vi "User Event LV2.vi"(11 "error in (no error)":errorcluster, 13 "LV2 Mode":T1=enum."Delete") -> (4 "Stop Val":refnum<user-event>, 15 "error out":errorcluster)   [LabVIEW 2020, in "I2C Controller Lib.lvlib"]
doc: "User events LV2 used to Create , Generate , Destroy User events . Can also be used as normal LV2"
uses:
  I2C Controller Lib.lvlib
  TypeDef/User LV2 Mode Select.ctl
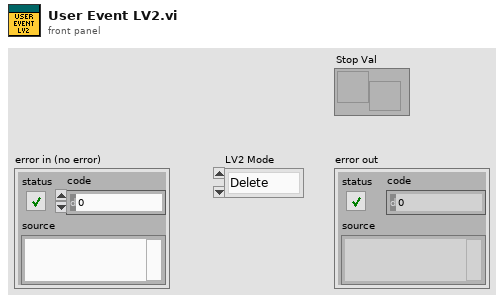
[diagram p1: front panel]
types:
  T1 = typedef "I2C Controller Lib.lvlib/User LV2 Mode Select.ctl" = enum16{"Create", "Delete", "Stop"}
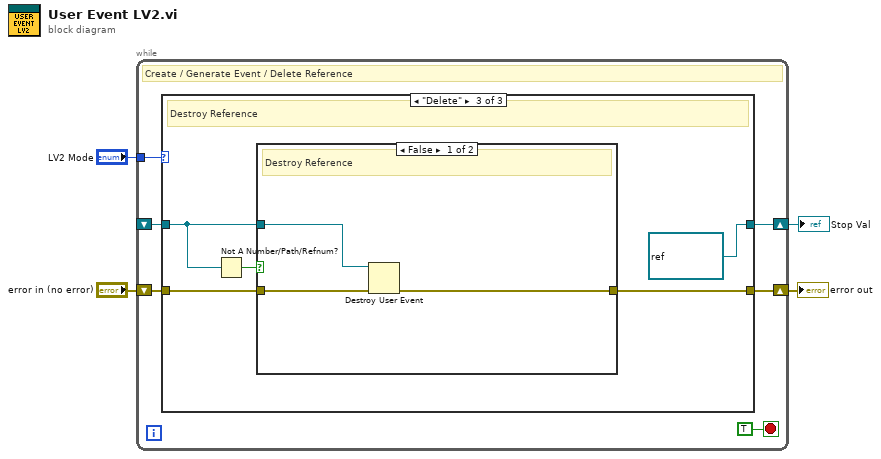
[diagram p0: block diagram]
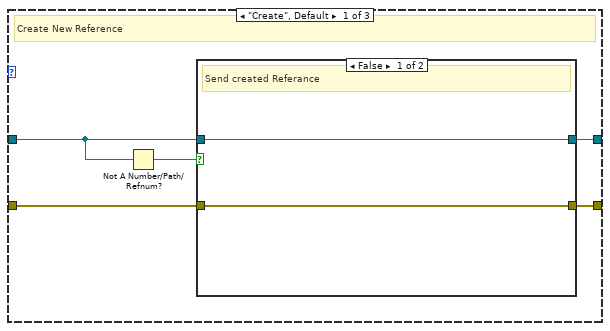
[diagram p2: hidden frame]
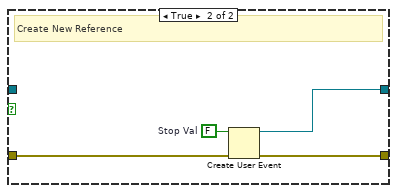
[diagram p3: hidden frame]
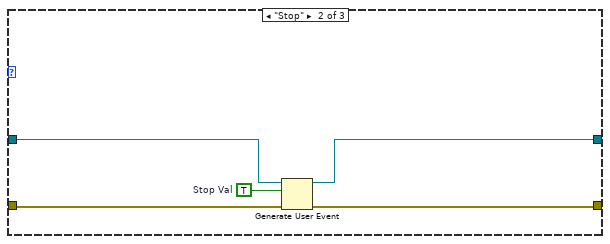
[diagram p4: hidden frame]
diagram:
  n1 = while {
    shift-right: [w7] -> w2
    shift-left: _ -> [w6]
    shift-right: [w8] -> w3
    shift-left: "error in (no error)" -> [w9]
    tunnel: "LV2 Mode" -> [w5]
    stop <- TRUE stop-if-true
    # "Create / Generate Event / Delete Reference"
    n2 = case shown="\"Delete\"" w5 {
      tunnel: w9 -> [w14 w24 w31]
      tunnel: [w13 w25 w30] -> w8
      tunnel: [w12 w23 refnum<user-event> refnum ("Stop Val")] -> w7
      tunnel: w6 -> [w11 w22 w27]
      frame "Create", Default {
        # "Create New Reference"
        n3 = Not A Number/Path/Refnum?(number/path/refnum=w11) -> (NaN/Path/Refnum?=w15:bool)
        n4 = case shown="False" w15 {
          tunnel: w14 -> [w17 w21]
          tunnel: [w17 w19] -> w13
          tunnel: [w16 w18] -> w12
          tunnel: w11 -> [w16 _]
          frame False {
            # "Send created Referance"
          }
          frame True {
            w20 = FALSE  # Stop Val
            # "Create New Reference"
            n5 = Create User Event(user event datatype=w20, error in=w21) -> (user event=w18:refnum<user-event>, error out=w19:errorcluster)
          }
        }
      }
      frame "Stop" {
        w26 = TRUE  # Stop Val
        n6 = Generate User Event(user event=w22, event data cluster=w26, error in=w24) -> (user event out=w23:refnum<user-event>, error out=w25:errorcluster)  [unwired: 1 in]
      }
      frame "Delete" {
        # "Destroy Reference"
        n7 = Not A Number/Path/Refnum?(number/path/refnum=w27) -> (NaN/Path/Refnum?=w29:bool)
        n8 = case shown="False" w29 {
          tunnel: w31 -> [w34 w35]
          tunnel: [w32 w35] -> w30
          tunnel: w27 -> [w33 _]
          frame False {
            # "Destroy Reference"
            n9 = Destroy User Event(user event=w33, error in=w34) -> (error out=w32:errorcluster)
          }
          frame True {
          }
        }
      }
    }
  }
  "error out" <- w3
  "Stop Val" <- w2
